vi "Dashboard Main.vi"() -> ()   [LabVIEW 2013]
uses:
  <vilib>/Rock Robotics/WPI/Camera/WPI_CameraWhite Balance Values.ctl
  <vilib>/Rock Robotics/WPI/Camera/WPI_CameraExposure Values.ctl
  <vilib>/Rock Robotics/WPI/Dashboard/WPI_DashboardLogging Global.vi
  <vilib>/Utility/config.llb/Write Key (String).vi
  <vilib>/Utility/config.llb/Write Key (I32).vi
  <vilib>/Utility/config.llb/NI_LVConfig.lvlib
panel:
  out "Image Message":string="Timeout in Camera Communications"
  in  "Rec Mode":enum32{"Stop", "Record", "Playback"}(radio)
  in  "Dashboard Tab":T1(tab)
  out "Battery":dbl(slide) scale=0.0..14.0
  in  "Camera Settings":T2={"Frame Rate"=30, "Compression"=30, "Size"=1} {"Frame Rate" scale=1.0..30.0; "Size" items=["640x480", "320x240", "160x120"]}
  out "Mode":T3(ring)=enum."Auto Disabled"
  out "Camera IP":string
  in  "DB Camera Config":bool
  out "fps":dbl format="%#.1g"
  out "Mbps 2":bool
  in  "Test Slider":dbl(slide) scale=0.0..100.0 scale format="%#_3g"
  in  "On/Off":bool caption="Solenoid"
  in  "Test Name":u16(ring) items=["Select the test to run...", "Example Test", "-------------------------------", "List of tests is built in robot code.", "Replace with your own automated tests."]
  in  "Test Tree":string(tree)
  in  "Motor":cluster{"Value":dbl, "Enable":bool} {"Value" scale=-1.0..1.0 scale format="%#_3g"}
  out "Progress":T4 {"Test Progress" scale=0.0..100.0}
  in  "Rev/Fwd":cluster{"Forward":bool, "Reverse":bool}
  in  "Test Ring":u16(ring) items=["Auto", "Fixed indoor", "Fixed outdoor 1", "Fixed outdoor 2", "Fixed fluorescent 1", "Fixed fluorescent 2", "Hold current"]
  out "Tree":string(tree)
  out "Camera Image":T5(plugin-control)
  in  "Enable":bool
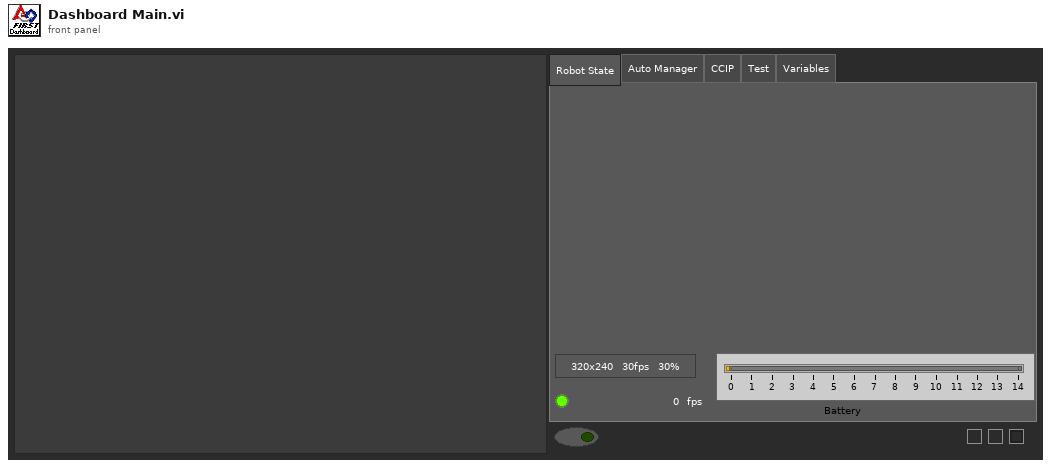
[diagram p1: front panel]
types:
  T1 = enum32{"Robot State", "Auto Manager", "CCIP", "Test", "Variables"}
  T2 = cluster{"Frame Rate":i32, "Compression":i32, "Size":u16}
  T3 = enum8{"Tele-Op Disabled", "Tele-Op Enabled", "Auto Disabled", "Auto Enabled", "Test Disabled", "Test Enabled", ""}
  T4 = cluster{"Test Progress":u8, "Test Progress Text":string}
  T5 = typedef "IMAQ Image.ctl" = refnum<image>
  T6 = typedef "WPI_CameraExposure Values.ctl" = enum16{"Auto", "Flicker-free 50 Hz", "Flicker-free 60 Hz", "Hold current"}
  T7 = typedef "WPI_CameraWhite Balance Values.ctl" = enum16{"Auto", "Fixed indoor", "Fixed outdoor 1", "Fixed outdoor 2", "Fixed fluorescent 1", "Fixed fluorescent 2", "Hold current"}
  T8 = enum32{"Drive", "Operation", "Auto", "Test", "Checklist", "Variables"}
  T9 = typedef "Image Type" = u32
  T10 = typedef "WPI_CameraDevRef.ctl" = cluster{"Camera Address":string, "CameraStatus":errorcluster, "Acquire Image Notifier":refnum<notifier>}
  T11 = cluster{"Digital Inputs":bool[], "Digital Outputs":bool[]}
  T12 = cluster{"Competition mode":bool, "Robot Link":bool, "Autonomous":bool, "Enabled":bool, "E-Stop":bool, "Simulated":bool, "TestMode":bool, "Docked Window":bool}
  T13 = typedef "WPI_CameraFrameRate.ctl" = u32
  T14 = cluster{"Score":sgl, "Fitted Circle":cluster{"Center":cluster{"X":sgl, "Y":sgl}, "Radius":dbl, "Circle Rect":cluster{"L":sgl, "T":sgl, "R":sgl, "B":sgl}, "Roundness":dbl, "SNR (dB)":dbl}, "Search Rect":cluster{"L":sgl, "T":sgl, "R":sgl, "B":sgl}, "Details":cluster{"Edge":sgl, "Area":sgl, "Circ":sgl, "Diam":sgl}}[]
  T15 = cluster{"Score":sgl, "Fitted Circle":cluster{"Center":cluster{"X":sgl, "Y":sgl}, "Radius":dbl, "Circle Rect":cluster{"L":sgl, "T":sgl, "R":sgl, "B":sgl}, "Roundness":dbl, "SNR (dB)":dbl}, "Search Rect":cluster{"L":sgl, "T":sgl, "R":sgl, "B":sgl}, "Details":cluster{"Edge":sgl, "Area":sgl, "Circ":sgl, "Diam":sgl}}
  T16 = typedef "NI_LVConfig.lvlib/Config Data RefNum.ctl" = refnum<k1>
  T17 = cluster{"Image Size":bool, "Image Type":bool, "Pixel Value":bool, "ROI Information":bool, "Zoom Factor":bool}
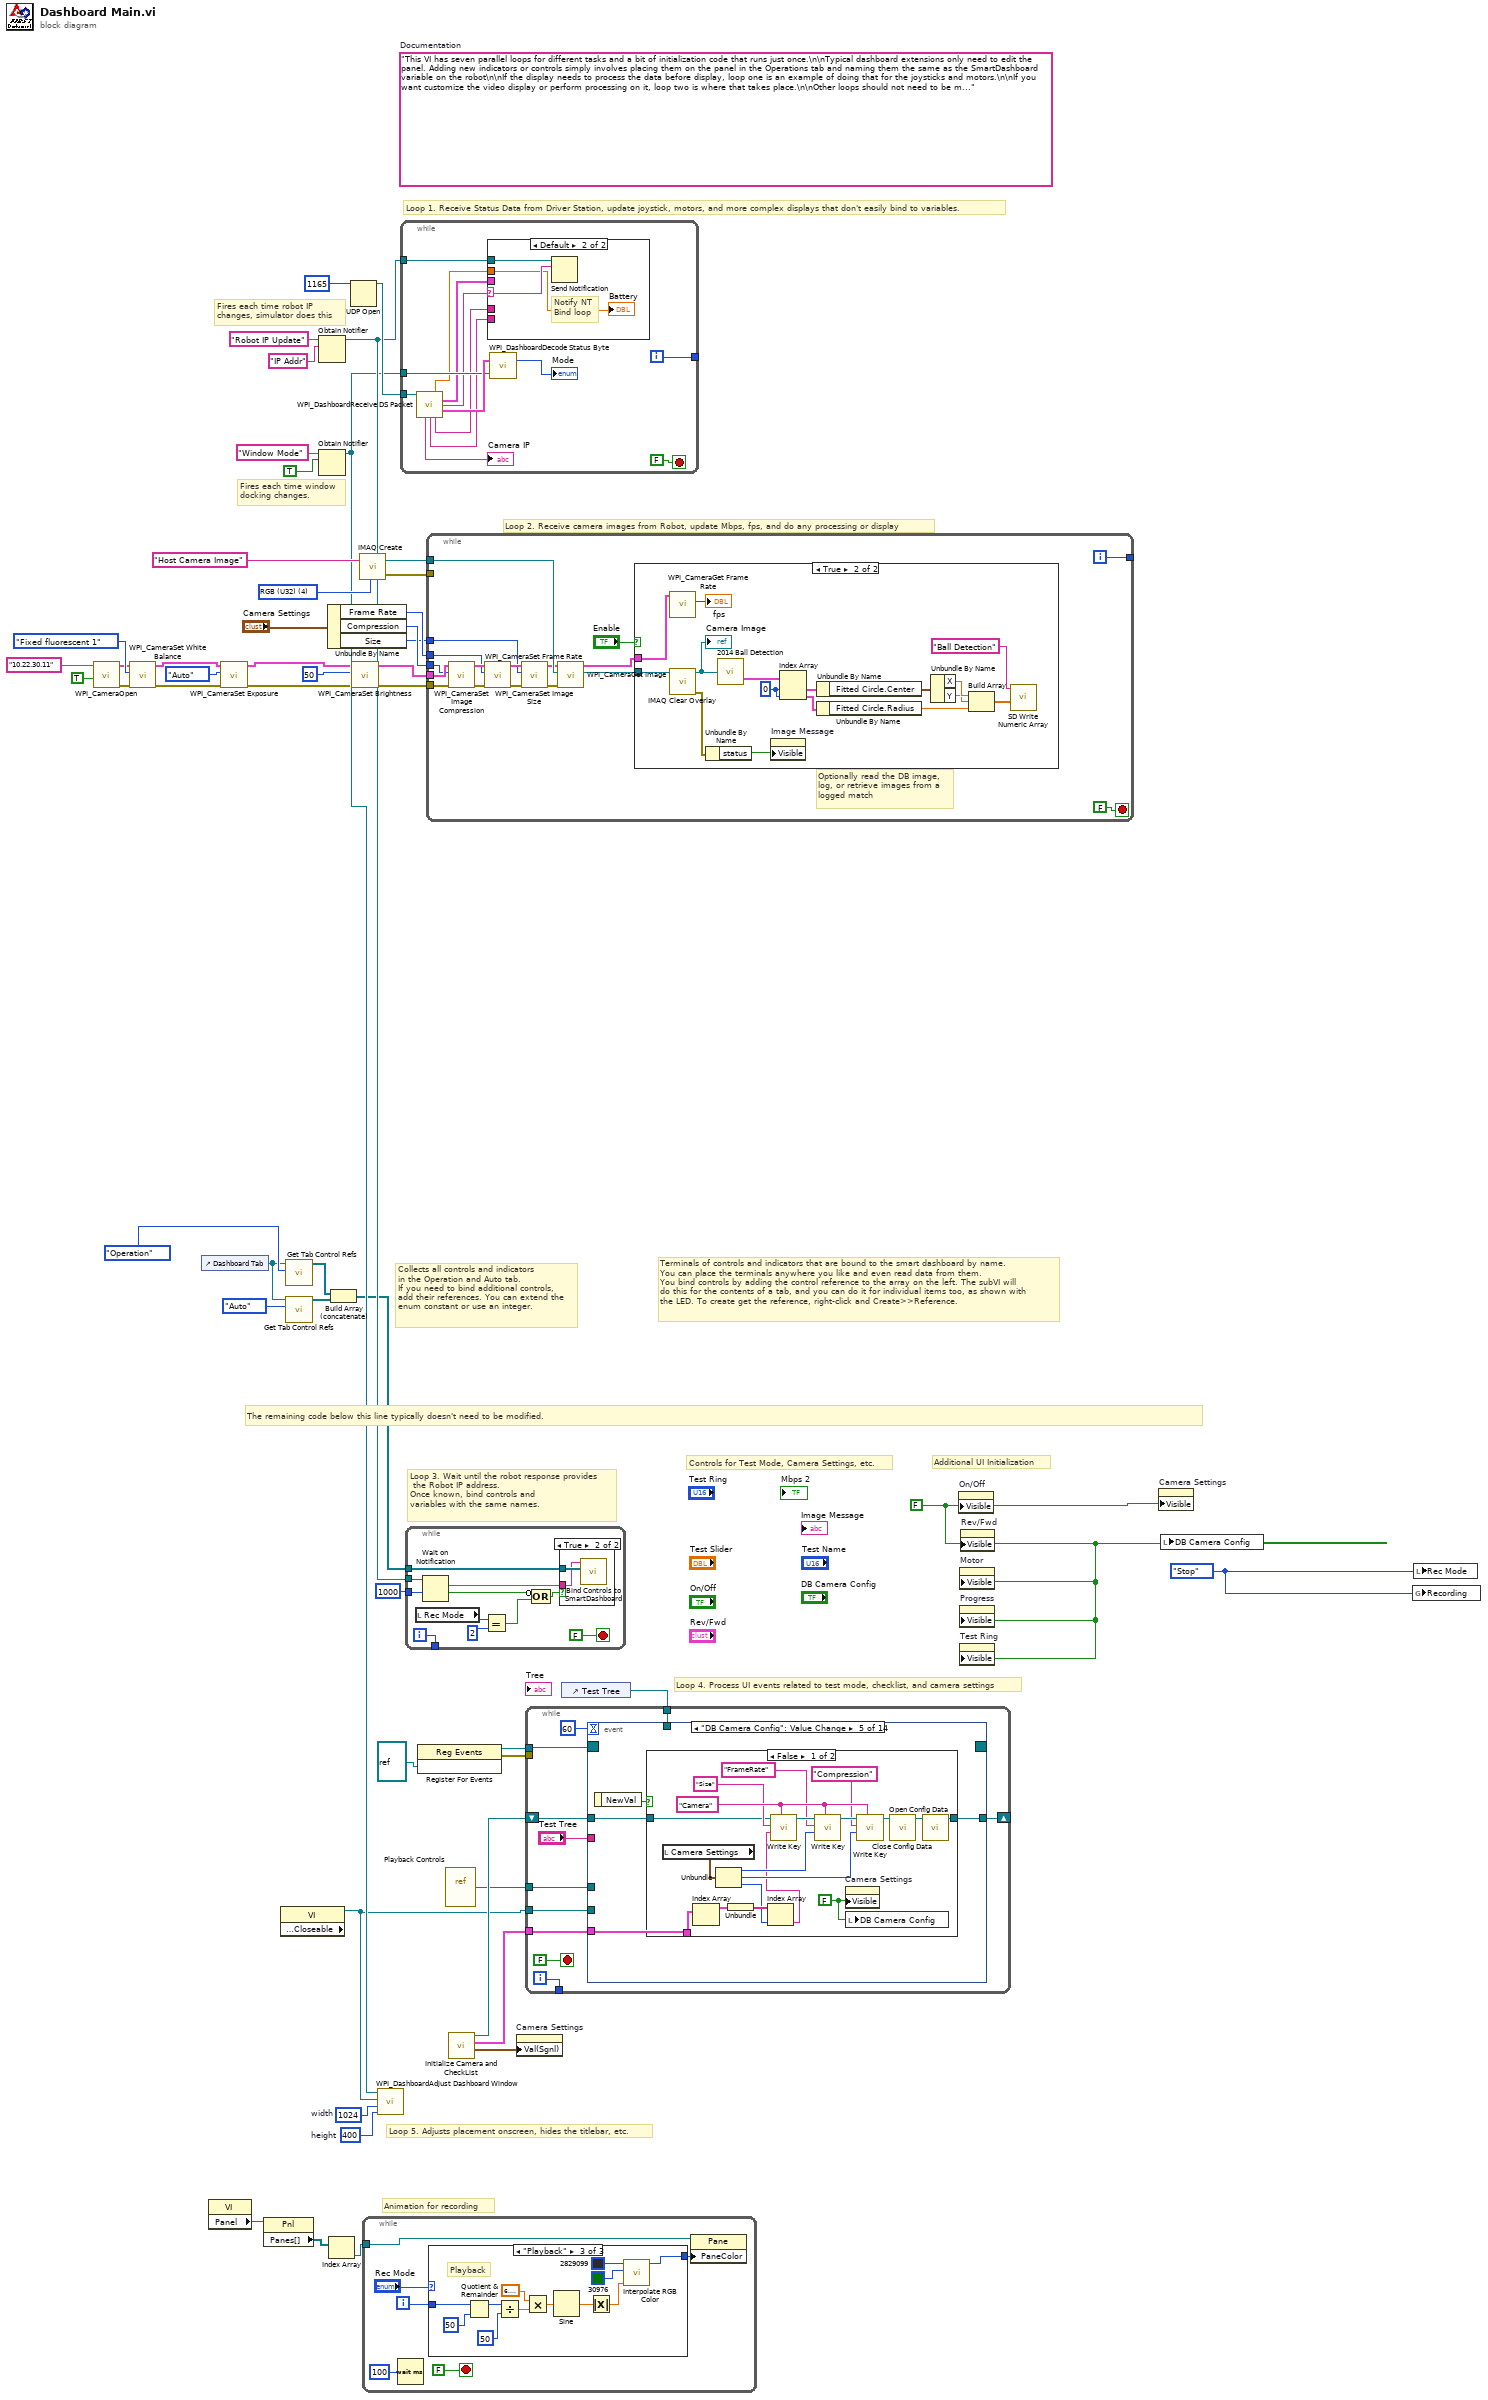
[diagram p0: block diagram]
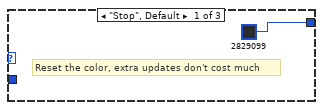
[diagram p2: hidden frame]
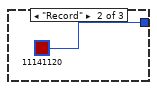
[diagram p3: hidden frame]
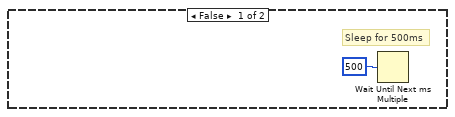
[diagram p5: hidden frame]
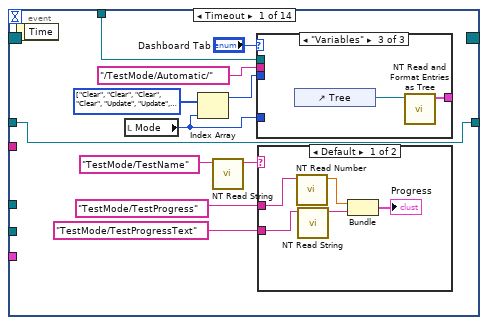
[diagram p6: hidden frame]
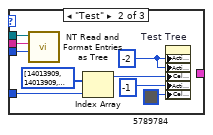
[diagram p8: hidden frame]
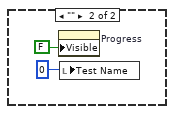
[diagram p9: hidden frame]
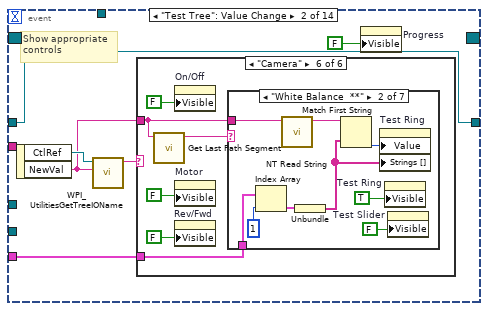
[diagram p10: hidden frame]
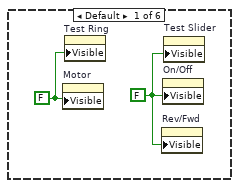
[diagram p11: hidden frame]
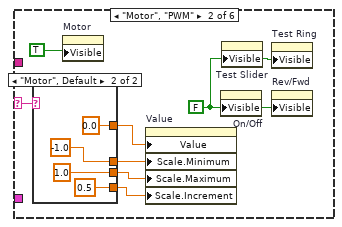
[diagram p12: hidden frame]
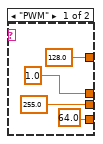
[diagram p13: hidden frame]
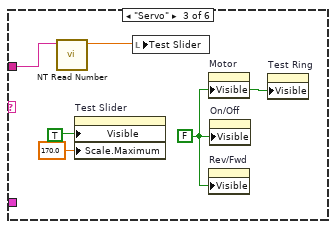
[diagram p14: hidden frame]
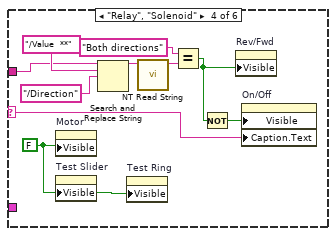
[diagram p15: hidden frame]
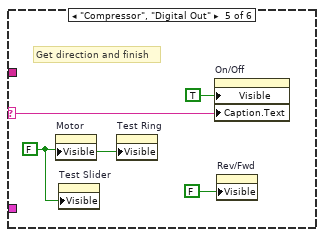
[diagram p16: hidden frame]
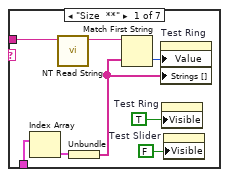
[diagram p17: hidden frame]
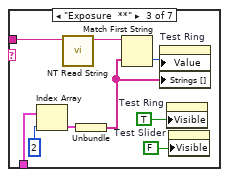
[diagram p18: hidden frame]
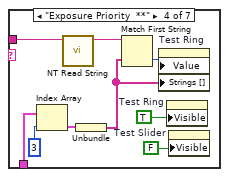
[diagram p19: hidden frame]
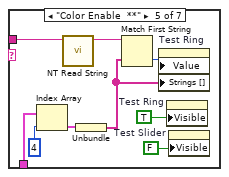
[diagram p20: hidden frame]
diagram:
  w24 = enum32{"Stop", "Record", "Playback"}."Stop" ("Rec Mode")
  w26 = 400  # height
  w27 = 1024  # width
  w40 = FALSE ("Visible")
  (unwired) "This VI has seven parallel loops for different tasks and a bit of initialization code that runs just once.\n\nTypical dashboard extensions only need to edit the panel. Adding new indicators or controls simply involves placing them on the panel in the Operations tab and naming them the same as the SmartDashboard variable on the robot\n\nIf the display needs to process the data before display, loop one is an example of doing that for the joysticks and motors.\n\nIf you want customize the video display or perform processing on it, loop two is where that takes place.\n\nOther loops should not need to be modified. They are pretty standard, and document the task they perform."  # Documentation
  w50 = T9 4 items=["Grayscale (U8)", "Grayscale (I16)", "Grayscale (SGL)", "Complex (CSG)", "RGB (U32)", "HSL (U32)", "RGB (U64)"] ("Image Type")
  # "Controls for Test Mode, Camera Settings, etc."
  # "Additional UI Initialization"
  # "Animation for recording"
  # "Fires each time robot IP\nchanges, simulator does this"
  # "Fires each time window\ndocking changes."
  # "Collects all controls and indicators\nin the Operation and Auto tab.\nIf you need to bind additional controls,\nadd their references. You can extend the\nenum constant or use an integer."
  # "The remaining code below this line typically doesn't need to be modified."
  # "Loop 4. Process UI events related to test mode, checklist, and camera settings"
  # "Terminals of controls and indicators that are bound to the smart dashboard by name.\nYou can place the terminals anywhere you like and even read data from them.\nYou bind controls by adding the control reference to the array on the left. The subVI will\ndo this for the contents of a tab, and you can do it for individual items too, as shown with\nthe LED. To create get the reference, right-click and Create>>Reference."
  # "Loop 3. Wait until the robot response provides\n the Robot IP address.\nOnce known, bind controls and\nvariables with the same names."
  # "Loop 5. Adjusts placement onscreen, hides the titlebar, etc."
  # "Loop 1. Receive Status Data from Driver Station, update joystick, motors, and more complex displays that don't easily bind to variables."
  # "Loop 2. Receive camera images from Robot, update Mbps, fps, and do any processing or display"
  n1 = call <vilib>:"WPI_CameraOpen.vi"("Disallow Simulation"=TRUE, "Camera Address"="10.22.30.11") -> ("error out"=w3:errorcluster, "CameraDevRef"=w4:T10)  [unwired: 1 in, 7 out]
  n2 = call <vilib>:"WPI_CameraSet White Balance.vi"("error in (no error)"=w3, "White Balance"=WPI_CameraWhite_Balance_Values."Fixed fluorescent 1", "CameraDevRef"=w4) -> ("error out"=w15:errorcluster, "CameraDevRef Out"=w14:T10)  [unwired: 7 out]
  n3 = control-ref of="Dashboard Tab"() -> (w22:refnum<vi>)
  n4 = property class="VI"() -> ("Panel"=w34:refnum<vi>)  [unwired: 2 in, 2 out]
  n5 = call <vilib>:"WPI_CameraSet Exposure.vi"("error in (no error)"=w15, "Exposure"=WPI_CameraExposure_Values."Auto", "CameraDevRef"=w14) -> ("error out"=w6:errorcluster, "CameraDevRef Out"=w9:T10)  [unwired: 7 out]
  n6 = property class="Pnl"(reference=w34) -> ("Panes[]"=w35:refnum<vi>[])  [unwired: 1 in, 2 out]
  n7 = property class="VI" props=["Front Panel.Closeable"]() -> (reference out=w23:refnum<vi>)  [unwired: 2 in, 2 out]
  n8 = call <vilib>:"Get Tab Control Refs.vi"("Page Index"=T8."Operation" ("Dashboard Tab"), "TabControl in"=w22) -> ("ControlsOnPage"=w20:refnum<vi>[])  [unwired: 9 in]
  n9 = call <vilib>:"Get Tab Control Refs.vi"("Page Index"=T8."Auto" ("Dashboard Tab"), "TabControl in"=w22) -> ("ControlsOnPage"=w21:refnum<vi>[])  [unwired: 9 in]
  n10 = Obtain Notifier(name (unnamed)="Robot IP Update", notification data type="IP Addr" ("name (unnamed)")) -> (notifier out=w44:refnum<notifier>)  [unwired: 2 in, 2 out]
  n11 = Obtain Notifier(name (unnamed)="Window Mode", notification data type=TRUE) -> (notifier out=w25:refnum<notifier>)  [unwired: 2 in, 2 out]
  n12 = Unbundle By Name("Camera Settings") -> ("Frame Rate"=w5:i32, "Compression"=w8:i32, "Size"=w2:u16)
  n13 = Index Array(array=w35) -> (element=w33:refnum<vi>)  [unwired: 1 in]
  n14 = Build Array (concatenate)(w20, w21) -> (w19:refnum<vi>[])
  n15 = UDP Open(11:u16 1165 ("port")) -> (port=w51:refnum<k16>)  [unwired: 2 in, 4 out]
  n16 = call <vilib>:"WPI_CameraSet Brightness.vi"("error in (no error)"=w6, "Brightness"=50, "CameraDevRef"=w9) -> ("error out"=w7:errorcluster, "CameraDevRef Out"=w10:T10)  [unwired: 7 out]
  n17 = call "IMAQ Create"("Image Name"="Host Camera Image", "Image Type"=w50) -> ("New Image"=w48:T5, "error out"=w47:errorcluster)  [unwired: 2 in, 1 out]
  n18 = while {
    tunnel: w33 -> [w54]
    i -> [w57]
    stop <- FALSE stop-if-true
    n19 = Wait (ms)(milliseconds to wait=u32 100) -> ()  [unwired: 1 out]
    n20 = case shown="\"Playback\"" "Rec Mode" {
      tunnel: w57 -> [_ _ w72]
      tunnel: [u32 2829099 ("Base Color") u32 11141120 ("Target Color") w61] -> w53
      frame "Stop", Default {
        # "Reset the color, extra updates don't cost much"
      }
      frame "Record" {
      }
      frame "Playback" {
        # "Playback"
        n21 = Quotient & Remainder(x=w72, y=u32 50 ("milliseconds to wait")) -> (x-y*floor(x/y)=w68:u32)  [unwired: 1 out]
        n22 = Divide(x=w68, y=u32 50 ("milliseconds to wait")) -> (x/y=w65:dbl)
        n23 = Multiply(x=6.283185307179586, y=w65) -> (x*y=w70:dbl)
        n24 = Sine(x=w70) -> (sin(x)=w69:dbl)
        n25 = Absolute Value(x=w69) -> (abs(x)=w62:dbl)
        n26 = call "Interpolate RGB Color.vi"("Proportion"=w62, "Target Color"=u32 30976, "Base Color"=u32 2829099) -> ("Result Color"=w61:u32)  [unwired: 8 in]
      }
    }
    n27 = property class="Pane"(reference=w54, "PaneColor"=w53) -> ()  [unwired: 1 in, 2 out]
  }
  n28 = call <vilib>:"WPI_DashboardAdjust Dashboard Window.vi"("height"=w26, "width"=w27, "reference in"=w23, "Notifier in"=w25) -> ()  [unwired: 8 in]
  n29 = while {
    tunnel: w51 -> [w83]
    tunnel: w44 -> [w78]
    tunnel: w25 -> [w82]
    tunnel: [w79] -> _
    i -> [w79]
    stop <- FALSE stop-if-true
    n30 = call <vilib>:"WPI_DashboardReceive DS Packet.vi"("Recv Socket"=w83) -> ("Battery"=w73:sgl, "Driver Station"=w74:T11, "Robot IP Address"=w77:string, "Status"=w84:T12, "Camera IP Address"=→"Camera IP":string, "Low Priority User Data"=w76:string, "High Priority User Data"=w75:string)  [unwired: 1 in, 7 out]
    n31 = case shown="Default" w77 {
      selector: w77 -> [_ w87]
      tunnel: w78 -> [_ w88]
      tunnel: w76 -> [_ _]
      tunnel: w75 -> [_ _]
      tunnel: w74 -> [_ _]
      tunnel: w73 -> [_ w86]
      frame "0.0.0.0" {
      }
      frame Default {
        # "Notify NT\nBind loop"
        n32 = Send Notification(notification=w87, notifier=w88) -> ()  [unwired: 1 in, 2 out]
        "Battery" <- w86
      }
    }
    n33 = call <vilib>:"WPI_DashboardDecode Status Byte.vi"("Window Mode Notifier"=w82, "Status"=w84) -> ("Mode"=→"Mode":T3)  [unwired: 1 out]
  }
  n34 = while {
    tunnel: w19 -> [w99]
    tunnel: w44 -> [w97]
    tunnel: [w95] -> _
    tunnel: u32 1000 ("milliseconds to wait") -> [w94]
    i -> [w95]
    stop <- FALSE stop-if-true
    n35 = local read "Rec Mode"() -> (w90:enum32{"Stop", "Record", "Playback"})
    n36 = Wait on Notification(notifier=w97, timeout in ms (-1)=w94) -> (notification=w96:string, timed out?=w92:bool)  [unwired: 2 in, 2 out]
    n37 = Equal?(x=w90, y=u16 2 ("Rec Mode")) -> (x = y?=w91:bool)
    n38 = Compound Arithmetic op=OR(invert w92, w91) -> (w93:bool)
    n39 = case shown="True" w93 {
      tunnel: w99 -> [_ w101]
      tunnel: w96 -> [_ w100]
      frame False {
      }
      frame True {
        n40 = call <vilib>:"Bind Controls to SmartDashboard.vi"("Bound Control Refs"=w101, "Server IP Address"=w100) -> ()  [unwired: 10 in]
      }
    }
  }
  n41 = register-events(refnum<vi> refnum) -> (reference out=w31:refnum<event-registration>, error out=w30:errorcluster)  [unwired: 2 in]
  n42 = while {
    tunnel: w48 -> [w115]
    tunnel: w47 -> [_]
    tunnel: [w117] -> _
    tunnel: w10 -> [w112]
    tunnel: w8 -> [w111]
    tunnel: w7 -> [w108]
    tunnel: w5 -> [w107]
    tunnel: w2 -> [w102]
    i -> [w117]
    stop <- FALSE stop-if-true
    # "Optionally read the DB image,\nlog, or retrieve images from a\nlogged match"
    n43 = call <vilib>:"WPI_CameraSet Image Compression.vi"("error in (no error)"=w108, "Compression"=w111, "CameraDevRef"=w112) -> ("error out"=w109:errorcluster, "CameraDevRef Out"=w110:T10)  [unwired: 7 out]
    n44 = call <vilib>:"WPI_CameraSet Frame Rate.vi"("error in (no error)"=w109, "Frame Rate (fps)"=w107, "CameraDevRef"=w110) -> ("error out"=w103:errorcluster, "CameraDevRef Out"=w104:T10)  [unwired: 7 out]
    n45 = call <vilib>:"WPI_CameraSet Image Size.vi"("error in (no error)"=w103, "Image Size"=w102, "CameraDevRef"=w104) -> ("error out"=w105:errorcluster, "CameraDevRef Out"=w106:T10)  [unwired: 7 out]
    n46 = call <vilib>:"WPI_CameraGet Image.vi"("error in (no error)"=w105, "Image"=w115, "CameraDevRef"=w106) -> ("Image Out"=w114:T5, "CameraDevRef Out"=w113:T10)  [unwired: 6 in, 1 out]
    n47 = case shown="True" "Enable" {
      tunnel: w114 -> [_ w133]
      tunnel: w113 -> [_ w131]
      frame False {
        # "Sleep for 500ms"
        n48 = Wait Until Next ms Multiple(millisecond multiple=u32 500) -> ()  [unwired: 1 out]
      }
      frame True {
        w120 = 0 ("index")
        n49 = call <vilib>:"WPI_CameraGet Frame Rate.vi"("CameraDevRef"=w131) -> ("Frame Rate (fps)"=→"fps":T13)  [unwired: 8 in, 2 out]
        n50 = call "IMAQ Clear Overlay"("Image"=w133) -> ("error out"=w134:errorcluster, "Image Out"=w130:T5)  [unwired: 2 in, 7 out]
        "Camera Image" <- w130
        n51 = Unbundle By Name(w134) -> ("status"=w135:bool)
        n52 = call "2014 Ball Detection.vi"("Image In"=w130) -> ("Ranked Objects"=w128:T14)  [unwired: 1 out]
        n53 = property on="Image Message" class="Str"("Visible"=w135) -> ()  [unwired: 2 in, 2 out]
        n54 = Index Array(array=w128, index #1=w120, index #2=w120) -> (element #1=w127:T15, element #2=w122:T15)
        n55 = Unbundle By Name(w127) -> ("Fitted Circle.Center"=w126:cluster{"X":sgl, "Y":sgl})
        n56 = Unbundle By Name(w122) -> ("Fitted Circle.Radius"=w121:dbl)
        n57 = Unbundle By Name(w126) -> ("X"=w125:sgl, "Y"=w124:sgl)
        n58 = Build Array(w125, w124, w121) -> (w123:dbl[])
        n59 = call <vilib>:"SD Write Numeric Array.vi"("Numeric Array"=w123, "Name"="Ball Detection") -> ()  [unwired: 8 in, 2 out]
      }
    }
  }
  n60 = vi-ref "Playback Controls.vi"() -> (w32:refnum<vi>)
  n61 = call "Initialize Camera and CheckList.vi"() -> ("Cluster"=w38:cluster{"value":i32, "value":i32, "index":i32}, "Array"=w39:cluster{string[]}[], "File Refnum"=w37:T16)  [unwired: 9 in]
  n62 = property on="Camera Settings" class="Clust (strict)"("Val(Sgnl)"=w38) -> ()  [unwired: 2 in, 2 out]
  n63 = control-ref of="Test Tree"() -> (w36:refnum<vi>)
  n64 = while {
    tunnel: w39 -> [w143]
    shift-right: [w142] -> _
    shift-left: w37 -> [w141]
    tunnel: [w140] -> _
    tunnel: w36 -> [w139]
    tunnel: w32 -> [w138]
    tunnel: w31 -> [w137]
    tunnel: w30 -> [_]
    tunnel: w23 -> [w136]
    i -> [w140]
    stop <- FALSE stop-if-true
    n65 = event shown="[4] \"DB Camera Config\": Value Change" {
      selector: w137 -> [_ _ _ _ _ _ _ _ _ _ _ _ _ _]
      dyn-events: [_ _ _ _ _ _ _ _ _ _ _ w357 _ _] -> _
      timeout: u32 60 ("milliseconds to wait") -> [_ _ _ _ _ _ _ _ _ _ _ _ _ _]
      tunnel: w139 -> [w153 _ _ _ _ _ _ _ _ _ _ _ _ _]
      tunnel: "Test Tree" -> [_ _ _ _ _ _ w326 w334 w336 w340 w348 _ _ _]
      tunnel: w143 -> [_ w177 _ _ w290 w320 _ _ _ _ _ _ _ _]
      tunnel: [w147 w176 w275 w280 w289 w313 w325 w332 w335 w339 w347 w359 w373 w374] -> w142
      tunnel: w141 -> [w147 w176 w275 w280 w288 w313 w325 w332 w335 w339 w347 w359 w373 w374]
      tunnel: w138 -> [_ _ _ _ _ _ _ _ _ _ _ w360 _ w377]
      tunnel: w136 -> [_ _ _ _ _ _ _ _ _ _ _ w355 _ _]
      event Timeout {
        w152 = enum16{"Update", "Clear"}[] [enum."Clear", enum."Clear", enum."Clear", enum."Clear", enum."Update", enum."Update", enum."Clear"] items=["Update", "Clear"]
        n66 = event-data() -> ()  [unwired: 1 in, 1 out]
        n67 = local read "Mode"() -> (w150:T3)
        n68 = Index Array(array=w152, index=w150) -> (element=w151:enum16{"Update", "Clear"})
        n69 = call <vilib>:"NT Read String.vi"("Name"="TestMode/TestName") -> ("String"=w156:string)  [unwired: 9 in, 1 out]
        n70 = case shown="\"Variables\"" "Dashboard Tab" {
          tunnel: w153 -> [_ w166 _]
          tunnel: "/TestMode/Automatic/" ("Name Pattern") -> [_ w165 _]
          tunnel: w151 -> [_ w164 _]
          tunnel: w150 -> [_ w162 _]
          tunnel: [_ _ w168] -> _
          frame "Auto Manager", Default {
          }
          frame "Test" {
            w161 = -2 ("Active Item:Row Number")
            n71 = call <vilib>:"NT Read and Format Entries as Tree.vi"("Operation"=w164, "Name Pattern"=w165, "Tree Refnum"=w166) -> ()  [unwired: 7 in, 2 out]
            n72 = Index Array(array=u32[] [14013909, 14013909, 14013909, 14013909, 14013909, 16777215, 14013909], index=w162) -> (element=w160:u32)
            n73 = property on="Test Tree" class="Tree (strict)"("Active Item Row Number"=w161, "ActiveColNum"=w161, "CellBG"=w160, "Active Item Row Number"=-1 ("Active Item:Row Number"), "CellBG"=u32 5789784 ("Color Box")) -> ()  [unwired: 2 in, 2 out]
          }
          frame "Variables" {
            n74 = control-ref of="Tree"() -> (w167:refnum<vi>)
            n75 = call <vilib>:"NT Read and Format Entries as Tree.vi"("Tree Refnum"=w167) -> ("Formatted Strings"=w168:cluster{"Name":string, "Value":string}[])  [unwired: 9 in, 1 out]
          }
        }
        n76 = case shown="Default" w156 {
          tunnel: "TestMode/TestProgress" ("Name") -> [w170 _]
          tunnel: "TestMode/TestProgressText" ("Name") -> [w169 _]
          frame Default {
            n77 = call <vilib>:"NT Read Number.vi"("Name"=w170) -> ("Numeric"=w171:dbl)  [unwired: 9 in, 1 out]
            n78 = call <vilib>:"NT Read String.vi"("Name"=w169) -> ("String"=w172:string)  [unwired: 9 in, 1 out]
            n79 = Bundle("Numeric"=w171, "String"=w172) -> (→"Progress":cluster{"Numeric":dbl, "String":string})  [unwired: 1 in]
          }
          frame "" {
            n80 = property on="Progress" class="Clust (strict)"("Visible"=FALSE) -> ()  [unwired: 2 in, 2 out]
            n81 = local write "Test Name"(u16 0) -> ()
          }
        }
      }
      event "Test Tree": Value Change {
        # "Show appropriate\ncontrols"
        n82 = event-data() -> ("CtlRef"=w180:refnum<vi>, "NewVal"=w178:string)  [unwired: 1 in]
        n83 = call <vilib>:"WPI_UtilitiesGetTreeIOName.vi"("NewVal"=w178, "TreeControl in"=w180) -> ("I/O Name"=w181:string)  [unwired: 9 in]
        n84 = case shown="\"Camera\"" w181 {
          selector: w181 -> [_ w188 _ w206 w215 _]
          tunnel: w178 -> [_ _ w203 w205 _ w222]
          tunnel: w177 -> [_ _ _ _ _ w221]
          frame Default {
            w183 = FALSE ("Visible")
            w182 = FALSE ("Visible")
            n85 = property on="Motor" class="Clust (strict)"("Visible"=w182) -> ()  [unwired: 2 in, 2 out]
            n86 = property on="Test Ring" class="Ring (strict)"("Visible"=w182) -> ()  [unwired: 2 in, 2 out]
            n87 = property on="Rev/Fwd" class="Clust (strict)"("Visible"=w183) -> ()  [unwired: 2 in, 2 out]
            n88 = property on="On/Off" class="Bool (strict)"("Visible"=w183) -> ()  [unwired: 2 in, 2 out]
            n89 = property on="Test Slider" class="Slide (strict)"("Visible"=w183) -> ()  [unwired: 2 in, 2 out]
          }
          frame "Motor", "PWM" {
            w189 = FALSE ("Visible")
            n90 = case shown="\"Motor\", Default" w188 {
              tunnel: [1.0 ("Value") -1.0 ("Value")] -> w187
              tunnel: [255.0 ("Value") 1.0 ("Value")] -> w186
              tunnel: [128.0 ("Value") 0.0 ("Value")] -> w185
              tunnel: [64.0 ("Value") 0.5 ("Value")] -> w184
              frame "PWM" {
              }
              frame "Motor", Default {
              }
            }
            n91 = property on="Motor" class="Clust (strict)"("Visible"=TRUE) -> ()  [unwired: 2 in, 2 out]
            n92 = property on="Value" class="Slide (strict)"("Value"=w185, "Scale.Minimum"=w187, "Scale.Maximum"=w186, "Scale.Increment"=w184) -> ()  [unwired: 2 in, 2 out]
            n93 = property on="On/Off" class="Bool (strict)"("Visible"=w189) -> ()  [unwired: 2 in, 2 out]
            n94 = property on="Test Slider" class="Slide (strict)"("Visible"=w189) -> ()  [unwired: 2 in, 2 out]
            n95 = property on="Test Ring" class="Ring (strict)"("Visible"=w189) -> ()  [unwired: 2 in, 2 out]
            n96 = property on="Rev/Fwd" class="Clust (strict)"("Visible"=w189) -> ()  [unwired: 2 in, 2 out]
          }
          frame "Servo" {
            w201 = FALSE ("Visible")
            n97 = call <vilib>:"NT Read Number.vi"("Name"=w203) -> ("Numeric"=w202:dbl)  [unwired: 9 in, 1 out]
            n98 = property on="Test Slider" class="Slide (strict)"("Visible"=TRUE, "Scale.Maximum"=170.0 ("Scale.Range:Maximum")) -> ()  [unwired: 2 in, 2 out]
            n99 = local write "Test Slider"(w202) -> ()
            n100 = property on="Motor" class="Clust (strict)"("Visible"=w201) -> ()  [unwired: 2 in, 2 out]
            n101 = property on="Rev/Fwd" class="Clust (strict)"("Visible"=w201) -> ()  [unwired: 2 in, 2 out]
            n102 = property on="On/Off" class="Bool (strict)"("Visible"=w201) -> ()  [unwired: 2 in, 2 out]
            n103 = property on="Test Ring" class="Ring (strict)"("Visible"=w201) -> ()  [unwired: 2 in, 2 out]
          }
          frame "Relay", "Solenoid" {
            w204 = FALSE ("Visible")
            n104 = property on="Motor" class="Clust (strict)"("Visible"=w204) -> ()  [unwired: 2 in, 2 out]
            n105 = property on="Test Slider" class="Slide (strict)"("Visible"=w204) -> ()  [unwired: 2 in, 2 out]
            n106 = Search and Replace String(input string=w205, search string="/Value  **", replace string="/Direction") -> (result string=w211:string)  [unwired: 5 in, 3 out]
            n107 = property on="Test Ring" class="Ring (strict)"("Visible"=w204) -> ()  [unwired: 2 in, 2 out]
            n108 = call <vilib>:"NT Read String.vi"("Name"=w211) -> ("String"=w209:string)  [unwired: 9 in, 1 out]
            n109 = Equal?(x="Both directions", y=w209) -> (x = y?=w207:bool)
            n110 = Not(x=w207) -> (.not. x?=w208:bool)
            n111 = property on="Rev/Fwd" class="Clust (strict)"("Visible"=w207) -> ()  [unwired: 2 in, 2 out]
            n112 = property on="On/Off" class="Bool (strict)"("Visible"=w208, "Caption.Text"=w206) -> ()  [unwired: 2 in, 2 out]
          }
          frame "Compressor", "Digital Out" {
            w214 = FALSE ("Visible")
            # "Get direction and finish"
            n113 = property on="Motor" class="Clust (strict)"("Visible"=w214) -> ()  [unwired: 2 in, 2 out]
            n114 = property on="Test Slider" class="Slide (strict)"("Visible"=w214) -> ()  [unwired: 2 in, 2 out]
            n115 = property on="Test Ring" class="Ring (strict)"("Visible"=w214) -> ()  [unwired: 2 in, 2 out]
            n116 = property on="On/Off" class="Bool (strict)"("Visible"=TRUE, "Caption.Text"=w215) -> ()  [unwired: 2 in, 2 out]
            n117 = property on="Rev/Fwd" class="Clust (strict)"("Visible"=FALSE) -> ()  [unwired: 2 in, 2 out]
          }
          frame "Camera" {
            n118 = call <vilib>:"Get Last Path Segment.vi"("String in"=w222) -> ("String out"=w223:string)  [unwired: 10 in]
            n119 = property on="On/Off" class="Bool (strict)"("Visible"=FALSE) -> ()  [unwired: 2 in, 2 out]
            n120 = property on="Motor" class="Clust (strict)"("Visible"=FALSE) -> ()  [unwired: 2 in, 2 out]
            n121 = property on="Rev/Fwd" class="Clust (strict)"("Visible"=FALSE) -> ()  [unwired: 2 in, 2 out]
            n122 = case shown="\"White Balance  **\"" w223 {
              tunnel: w222 -> [w229 w238 w247 w256 w265 _ w271]
              tunnel: w221 -> [w227 w235 w244 w253 w262 _ _]
              frame "Size  **" {
                n123 = Index Array(array=w227) -> (element=w226:cluster{string[]})  [unwired: 1 in]
                n124 = call <vilib>:"NT Read String.vi"("Name"=w229) -> ("String"=w228:string)  [unwired: 9 in, 1 out]
                n125 = Unbundle(w226) -> (w224:string[])
                n126 = Match First String(2:w224, 3:w228) -> (0:w225:i32)  [unwired: 1 out]
                n127 = property on="Test Ring" class="Ring (strict)"("Value"=w225, "Strings []"=w224) -> ()  [unwired: 2 in, 2 out]
                n128 = property on="Test Ring" class="Ring (strict)"("Visible"=TRUE) -> ()  [unwired: 2 in, 2 out]
                n129 = property on="Test Slider" class="Slide (strict)"("Visible"=FALSE) -> ()  [unwired: 2 in, 2 out]
              }
              frame "White Balance  **" {
                n130 = Index Array(array=w235, index=1) -> (element=w236:cluster{string[]})
                n131 = call <vilib>:"NT Read String.vi"("Name"=w238) -> ("String"=w237:string)  [unwired: 9 in, 1 out]
                n132 = Unbundle(w236) -> (w233:string[])
                n133 = Match First String(2:w233, 3:w237) -> (0:w232:i32)  [unwired: 1 out]
                n134 = property on="Test Ring" class="Ring (strict)"("Value"=w232, "Strings []"=w233) -> ()  [unwired: 2 in, 2 out]
                n135 = property on="Test Ring" class="Ring (strict)"("Visible"=TRUE) -> ()  [unwired: 2 in, 2 out]
                n136 = property on="Test Slider" class="Slide (strict)"("Visible"=FALSE) -> ()  [unwired: 2 in, 2 out]
              }
              frame "Exposure  **" {
                n137 = Index Array(array=w244, index=2) -> (element=w245:cluster{string[]})
                n138 = call <vilib>:"NT Read String.vi"("Name"=w247) -> ("String"=w246:string)  [unwired: 9 in, 1 out]
                n139 = Unbundle(w245) -> (w241:string[])
                n140 = Match First String(2:w241, 3:w246) -> (0:w242:i32)  [unwired: 1 out]
                n141 = property on="Test Ring" class="Ring (strict)"("Value"=w242, "Strings []"=w241) -> ()  [unwired: 2 in, 2 out]
                n142 = property on="Test Ring" class="Ring (strict)"("Visible"=TRUE) -> ()  [unwired: 2 in, 2 out]
                n143 = property on="Test Slider" class="Slide (strict)"("Visible"=FALSE) -> ()  [unwired: 2 in, 2 out]
              }
              frame "Exposure Priority  **" {
                n144 = Index Array(array=w253, index=3) -> (element=w254:cluster{string[]})
                n145 = call <vilib>:"NT Read String.vi"("Name"=w256) -> ("String"=w255:string)  [unwired: 9 in, 1 out]
                n146 = Unbundle(w254) -> (w250:string[])
                n147 = Match First String(2:w250, 3:w255) -> (0:w251:i32)  [unwired: 1 out]
                n148 = property on="Test Ring" class="Ring (strict)"("Value"=w251, "Strings []"=w250) -> ()  [unwired: 2 in, 2 out]
                n149 = property on="Test Ring" class="Ring (strict)"("Visible"=TRUE) -> ()  [unwired: 2 in, 2 out]
                n150 = property on="Test Slider" class="Slide (strict)"("Visible"=FALSE) -> ()  [unwired: 2 in, 2 out]
              }
              frame "Color Enable  **" {
                n151 = Index Array(array=w262, index=4) -> (element=w263:cluster{string[]})
                n152 = call <vilib>:"NT Read String.vi"("Name"=w265) -> ("String"=w264:string)  [unwired: 9 in, 1 out]
                n153 = Unbundle(w263) -> (w259:string[])
                n154 = Match First String(2:w259, 3:w264) -> (0:w260:i32)  [unwired: 1 out]
                n155 = property on="Test Ring" class="Ring (strict)"("Value"=w260, "Strings []"=w259) -> ()  [unwired: 2 in, 2 out]
                n156 = property on="Test Ring" class="Ring (strict)"("Visible"=TRUE) -> ()  [unwired: 2 in, 2 out]
                n157 = property on="Test Slider" class="Slide (strict)"("Visible"=FALSE) -> ()  [unwired: 2 in, 2 out]
              }
              frame Default {
                n158 = property on="Test Ring" class="Ring (strict)"("Visible"=FALSE) -> ()  [unwired: 2 in, 2 out]
                n159 = property on="Test Slider" class="Slide (strict)"("Visible"=FALSE) -> ()  [unwired: 2 in, 2 out]
              }
              frame "Brightness  **", "Color Level  **", "Compression  **", "FPS  **", "Sharpness  **" {
                n160 = call <vilib>:"NT Read Number.vi"("Name"=w271) -> ("Numeric"=w270:dbl)  [unwired: 9 in, 1 out]
                n161 = local write "Test Slider"(w270) -> ()
                n162 = property on="Test Slider" class="Slide (strict)"("Visible"=TRUE, "Scale.Maximum"=100.0 ("Scale.Range:Maximum")) -> ()  [unwired: 2 in, 2 out]
                n163 = property on="Test Ring" class="Ring (strict)"("Visible"=FALSE) -> ()  [unwired: 2 in, 2 out]
              }
            }
          }
        }
        n164 = property on="Progress" class="Clust (strict)"("Visible"=FALSE) -> ()  [unwired: 2 in, 2 out]
      }
      event "Test Name": Mouse Enter {
        # "Populate the ring with the list of tests"
        n165 = event-data() -> ()  [unwired: 1 in, 1 out]
        n166 = call <vilib>:"NT Read String Array.vi"("Name"="TestMode/TestList") -> ("String Array"=w279:string[])  [unwired: 9 in, 1 out]
        n167 = Build Array (concatenate)("Select the test to run...", w279) -> (w278:string[])
        n168 = property on="Test Name" class="Ring (strict)"("Strings []"=w278) -> ()  [unwired: 2 in, 2 out]
      }
      event "Test Name": Value Change {
        w281 = FALSE ("Visible")
        # "Tell the robot the test name to run"
        n169 = event-data() -> ("NewVal"=w285:u16)  [unwired: 1 in]
        n170 = property on="Test Name" class="Ring (strict)"() -> ("Strings []"=w286:string[])  [unwired: 2 in, 2 out]
        n171 = local write "Progress"(T4 {"Test Progress"=0, "Test Progress Text"=""} ("Progress")) -> ()
        n172 = Index Array(array=w286, index=w285) -> (element=w284:string)
        n173 = call <vilib>:"NT Write String.vi"("String"=w284, "Name"="TestMode/TestName") -> ()  [unwired: 9 in, 1 out]
        n174 = property on="Progress" class="Clust (strict)"("Visible"=TRUE) -> ()  [unwired: 2 in, 2 out]
        n175 = property on="Motor" class="Clust (strict)"("Visible"=w281) -> ()  [unwired: 2 in, 2 out]
        n176 = property on="Test Slider" class="Slide (strict)"("Visible"=w281) -> ()  [unwired: 2 in, 2 out]
        n177 = property on="On/Off" class="Bool (strict)"("Visible"=w281) -> ()  [unwired: 2 in, 2 out]
        n178 = property on="Rev/Fwd" class="Clust (strict)"("Visible"=w281) -> ()  [unwired: 2 in, 2 out]
        n179 = property on="Test Ring" class="Ring (strict)"("Visible"=w281) -> ()  [unwired: 2 in, 2 out]
      }
      event "DB Camera Config": Value Change {
        n180 = event-data() -> ("NewVal"=w291:bool)  [unwired: 1 in]
        n181 = case shown="False" w291 {
          tunnel: w290 -> [w300 _]
          tunnel: [w293 w311] -> w289
          tunnel: w288 -> [w292 w311]
          frame False {
            w307 = "Camera"
            w310 = FALSE ("Visible")
            n182 = local read "Camera Settings"() -> (w299:T2)
            n183 = Index Array(array=w300) -> (element=w303:cluster{string[]})  [unwired: 1 in]
            n184 = Unbundle(w299) -> ("Frame Rate"=w298:i32, "Compression"=w297:i32, "Size"=w301:u16)
            n185 = Unbundle(w303) -> (w302:string[])
            n186 = Index Array(array=w302, index=w301) -> (element=w296:string)
            n187 = call-poly <vilib>:"Write Key.vi"("section"=w307, "value"=w296, "key"="Size", "refnum"=w292) -> ("refnum out"=w309:T16)  [unwired: 2 in, 5 out]
            n188 = call-poly <vilib>:"Write Key.vi"("section"=w307, "value"=w298, "key"="FrameRate", "refnum"=w309) -> ("refnum out"=w308:T16)  [unwired: 1 in, 6 out]
            n189 = property on="Camera Settings" class="Clust (strict)"("Visible"=w310) -> ()  [unwired: 2 in, 2 out]
            n190 = local write "DB Camera Config"(w310) -> ()
            n191 = call-poly <vilib>:"Write Key.vi"("section"=w307, "value"=w297, "key"="Compression", "refnum"=w308) -> ("refnum out"=w294:T16)  [unwired: 1 in, 6 out]
            n192 = call <vilib>:"Close Config Data.vi"("refnum"=w294) -> ("file path"=w295:path)  [unwired: 2 in, 8 out]
            n193 = call <vilib>:"Open Config Data.vi"("configuration file path"=w295) -> ("refnum"=w293:T16)  [unwired: 8 in, 2 out]
          }
          frame True {
            n194 = property on="Camera Settings" class="Clust (strict)"("Visible"=TRUE) -> ()  [unwired: 2 in, 2 out]
          }
        }
      }
      event "Camera Settings": Value Change {
        n195 = event-data() -> ("NewVal"=w324:T2)  [unwired: 1 in]
        n196 = Index Array(array=w320) -> (element=w319:cluster{string[]})  [unwired: 1 in]
        n197 = Unbundle(w324) -> ("Frame Rate"=w315:i32, "Compression"=w314:i32, "Size"=w317:u16)
        n198 = Unbundle(w319) -> (w318:string[])
        n199 = Index Array(array=w318, index=w317) -> (element=w316:string)
        n200 = Format Into String(format string="%s   %dfps   %d%%", w316, w315, w314) -> (resulting string=w321:string)  [unwired: 2 in, 1 out]
        n201 = Build Array(w321) -> (w322:string[])
        n202 = property on="DB Camera Config" class="Bool (strict)"("Strings [4]"=w322) -> ()  [unwired: 2 in, 2 out]
      }
      event "Motor.Enable": Value Change {
        n203 = event-data() -> ("NewVal"=w330:bool)  [unwired: 1 in]
        n204 = Unbundle("Motor") -> ("Value"=w329:dbl)  [unwired: 1 out]
        n205 = Select(t=w329, s=w330, f=0.0) -> (s? t:f=w327:dbl)
        n206 = call <vilib>:"NT Write Number.vi"("Numeric"=w327, "Name"=w326) -> ()  [unwired: 9 in, 1 out]
      }
      event "Test Slider": Value Change {
        n207 = event-data() -> ("NewVal"=w333:dbl)  [unwired: 1 in]
        n208 = call <vilib>:"NT Write Number.vi"("Numeric"=w333, "Name"=w334) -> ()  [unwired: 9 in, 1 out]
      }
      event "On/Off": Value Change {
        n209 = event-data() -> ("NewVal"=w338:bool)  [unwired: 1 in]
        n210 = Boolean To (0,1)(Boolean=w338) -> (0, 1=w337:i16)
        n211 = call <vilib>:"NT Write Number.vi"("Numeric"=w337, "Name"=w336) -> ()  [unwired: 9 in, 1 out]
      }
      event "Rev/Fwd": Value Change {
        n212 = event-data() -> ("NewVal.Forward"=w346:bool, "NewVal.Reverse"=w345:bool)  [unwired: 1 in]
        n213 = Boolean To (0,1)(Boolean=w346) -> (0, 1=w342:i16)
        n214 = Boolean To (0,1)(Boolean=w345) -> (0, 1=w344:i16)
        n215 = Negate(x=w344) -> (-x=w343:i16)
        n216 = Add(x=w342, y=w343) -> (x+y=w341:i16)
        n217 = call <vilib>:"NT Write Number.vi"("Numeric"=w341, "Name"=w340) -> ()  [unwired: 9 in, 1 out]
      }
      event "Test Ring": Value Change {
        n218 = event-data() -> ("NewVal"=w350:u16)  [unwired: 1 in]
        n219 = property on="Test Ring" class="Ring (strict)"() -> ("Strings []"=w351:string[])  [unwired: 2 in, 2 out]
        n220 = Index Array(array=w351, index=w350) -> (element=w349:string)
        n221 = call <vilib>:"NT Write String.vi"("String"=w349, "Name"=w348) -> ()  [unwired: 9 in, 1 out]
      }
      event "Rec Mode": Value Change {
        # "Update globals for recording mode and path to read log from.\nClear when logging and let NetworkTables set path for vision to\nuse."
        n222 = event-data() -> ("NewVal"=w361:enum32{"Stop", "Record", "Playback"})  [unwired: 1 in]
        n223 = global write "WPI_DashboardLogging Global.vi" "Logging Filename"(path "") -> ()
        n224 = case shown="\"Stop\", \"Record\"" w361 {
          tunnel: w360 -> [_ w363 w371]
          tunnel: [_ _ w370] -> w357
          tunnel: [_ _ w369] -> _
          tunnel: w355 -> [_ _ w367]
          tunnel: cluster{i32, i32} {-250, 170} -> [_ _ w366]
          tunnel: [_ _ T17 {"Image Size"=TRUE, "Image Type"=TRUE, "Pixel Value"=TRUE, "ROI Information"=TRUE, "Zoom Factor"=FALSE} ("Image Information Shown:All Elements")] -> w353
          tunnel: [_ _ TRUE ("Zoom Factor")] -> w352
          frame Default {
          }
          frame "Stop", "Record" {
            # "Place Window too"
            n225 = invoke class="VI" method="FP.Close"(reference=w363) -> (reference out=w362:refnum<vi>)  [unwired: 2 in, 2 out]
            n226 = invoke class="VI" method="Abort VI"(reference=w362) -> ()  [unwired: 2 in, 3 out]
          }
          frame "Playback" {
            n227 = call "Open Playback Panel.vi"("Offset"=w366, "DB VI Ref"=w367, "Playback in"=w371) -> ("Playback out"=w368:refnum<vi>)  [unwired: 8 in]
            n228 = register-events(w368) -> (reference out=w370:refnum<event-registration>, error out=w369:errorcluster)  [unwired: 2 in]
          }
        }
        n229 = global write "WPI_DashboardLogging Global.vi" "Recording"(w361) -> ()
        n230 = property on="Camera Image" class="ImageControl"("Image Information Shown"=w353, "Image Information Visible"=w352) -> ()  [unwired: 2 in, 2 out]
        n231 = call <vilib>:"WPI_DashboardNT Log FieldName Cache.vi"("Operation"=enum16{"Lookup/Add", "Index", "Clear"}."Clear") -> ()  [unwired: 8 in, 3 out]
      }
      event Panel Close {
        w372 = enum32{"Stop", "Record", "Playback"}."Stop" ("Rec Mode")
        n232 = event-data() -> ()  [unwired: 1 in, 4 out]
        n233 = local write "Rec Mode"(w372) -> ()
        n234 = global write "WPI_DashboardLogging Global.vi" "Recording"(w372) -> ()
      }
      event Panel Close {
        # "Abort playback window and ourself"
        n235 = event-data() -> ()  [unwired: 1 in, 4 out]
        n236 = invoke class="VI" method="FP.Close"(reference=w377) -> (reference out=w376:refnum<vi>)  [unwired: 2 in, 2 out]
        n237 = invoke class="VI" method="Abort VI"(reference=w376) -> (error out=w375:errorcluster)  [unwired: 2 in, 2 out]
        n238 = invoke class="VI" method="Abort VI"(error in=w375) -> ()  [unwired: 2 in, 3 out]
      }
    }
  }
  n239 = property on="On/Off" class="Bool (strict)"("Visible"=w40) -> ()  [unwired: 2 in, 2 out]
  n240 = property on="Motor" class="Clust (strict)"("Visible"=w40) -> ()  [unwired: 2 in, 2 out]
  n241 = property on="Progress" class="Clust (strict)"("Visible"=w40) -> ()  [unwired: 2 in, 2 out]
  n242 = property on="Test Ring" class="Ring (strict)"("Visible"=w40) -> ()  [unwired: 2 in, 2 out]
  n243 = property on="Rev/Fwd" class="Clust (strict)"("Visible"=w40) -> ()  [unwired: 2 in, 2 out]
  n244 = property on="Camera Settings" class="Clust (strict)"("Visible"=w40) -> ()  [unwired: 2 in, 2 out]
  n245 = local write "DB Camera Config"(w40) -> ()
  n246 = global write "WPI_DashboardLogging Global.vi" "Recording"(w24) -> ()
  n247 = local write "Rec Mode"(w24) -> ()
